vi "refnums.vi"() -> ()   [LabVIEW 2019]
doc: "This global variable contains refnum names. All refnum names are set in Begin."
panel:
  out "Turret_Simulator_Servo":string
  out "Number_of_LEDs":u16
  out "Swerve_2_Shifter":string
  out "Swerve_1_Shifter":string
  out "Swerve_0_Shifter":string
  out "IMU_Talon":string
  out "Swerve_3_Shifter":string
  out "LIDAR":string
  out "Intake_Deploy":string
  out "Intake":string
  out "Pressure_Transducer":string
  out "Joystick_Manipulator":string
  out "Swerve_3_Pot":string
  out "Swerve_2_Pot":string
  out "Swerve_1_Pot":string
  out "Swerve_0_Pot":string
  out "Swerve_3_Azimuth":string
  out "Swerve_2_Azimuth":string
  out "IMU_0":string
  out "Joystick_Driver":string
  out "Compressor":string
  out "Swerve_1_Azimuth":string
  out "Swerve_0_Azimuth":string
  out "Swerve_3_Drive":string
  out "Swerve_2_Drive":string
  out "Swerve_1_Drive":string
  out "Swerve_0_Drive":string
  # "--pressure management--"
  # "--miscellaneous--"
  # "--intake subsystem--"
  # "--driver station--"
  # "--drive subsystem--"
  # "--other sensors--"
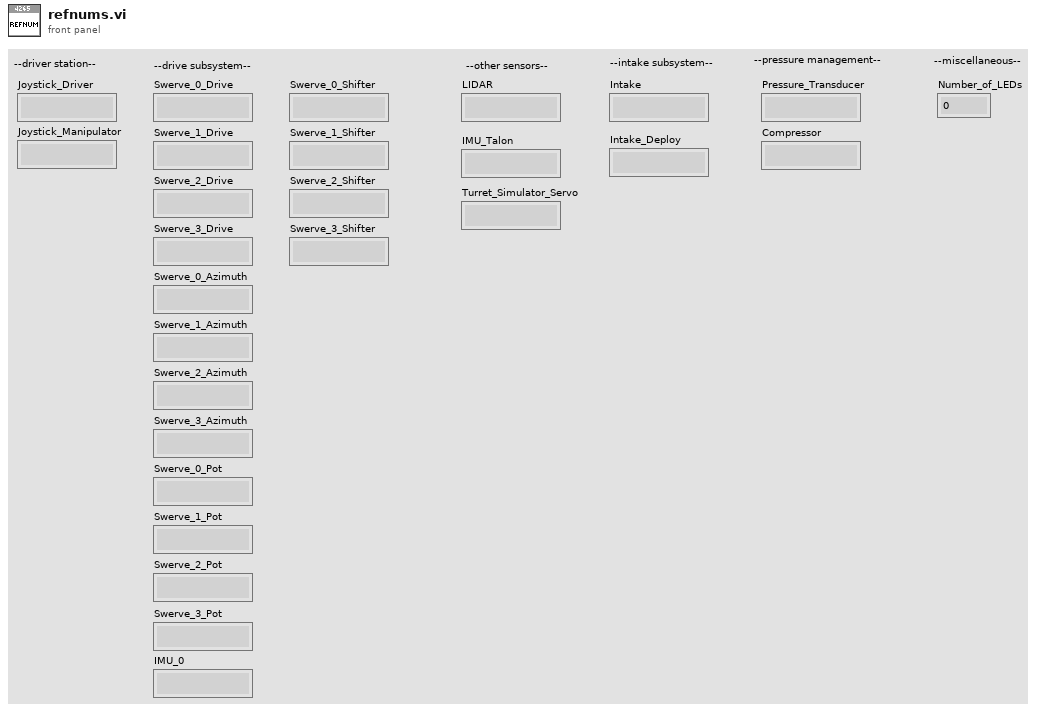
[diagram p1: front panel]
diagram:
